vi "GatheringSerialPortNames.vi"() -> (1 "name":string)   [LabVIEW 2016]
panel:
  in  "done":bool
  in  "Name":string
  in  "Refresh":bool
  in  "Name It":bool
  in  "Ports":i32(listbox)
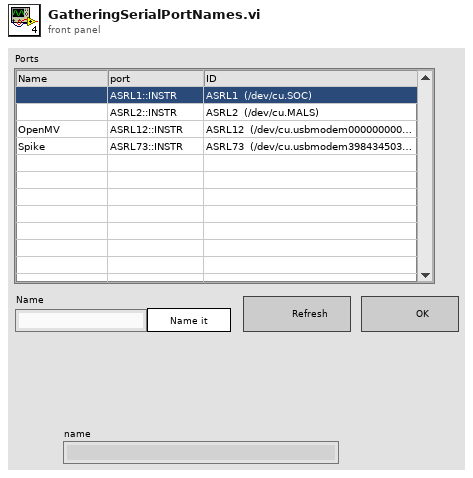
[diagram p1: front panel]
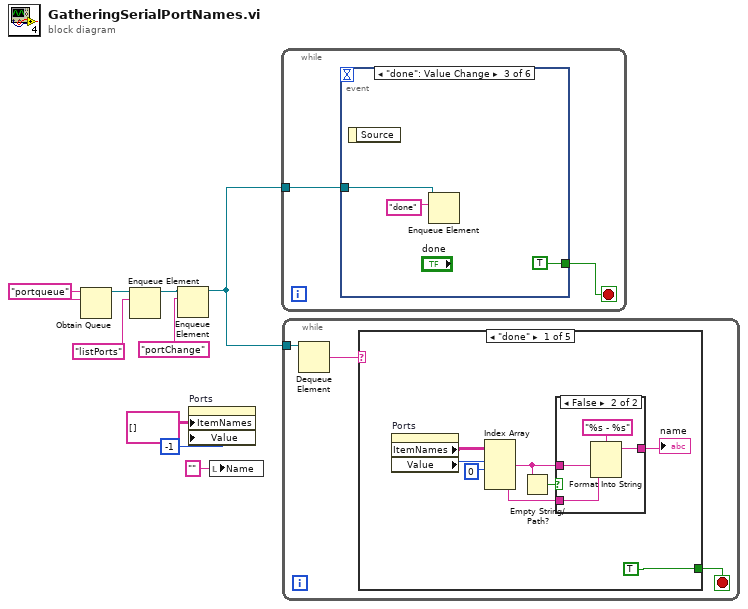
[diagram p0: block diagram]
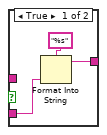
[diagram p2: hidden frame]
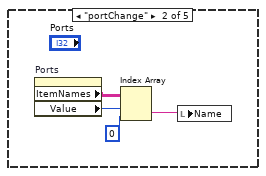
[diagram p3: hidden frame]
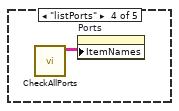
[diagram p5: hidden frame]
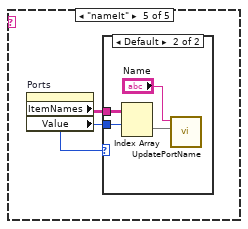
[diagram p6: hidden frame]
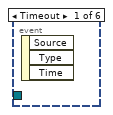
[diagram p8: hidden frame]
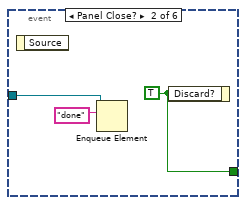
[diagram p9: hidden frame]
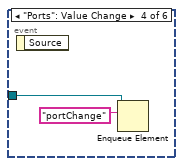
[diagram p10: hidden frame]
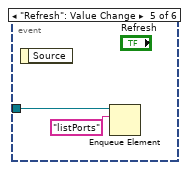
[diagram p11: hidden frame]
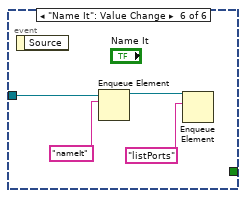
[diagram p12: hidden frame]
diagram:
  w7 = "portqueue" ("name (unnamed)")
  n1 = Obtain Queue(name (unnamed)=w7, element data type=w7) -> (queue out=w9:refnum<queue>)  [unwired: 3 in, 2 out]
  n2 = Enqueue Element(queue=w9, element="listPorts") -> (queue out=w5:refnum<queue>)  [unwired: 2 in, 2 out]
  n3 = Enqueue Element(queue=w5, element="portChange") -> (queue out=w4:refnum<queue>)  [unwired: 2 in, 2 out]
  n4 = property on="Ports" class="MCListbox (strict)"("ItemNames"=string[][] [] ("Item Names"), "Value"=-1 ("Ports")) -> ()  [unwired: 2 in, 2 out]
  n5 = local write "Name"("" ("Name")) -> ()
  n6 = while {
    tunnel: w4 -> [w10]
    stop <- w11 stop-if-true
    n7 = event shown="[2] \"done\": Value Change" {
      selector: _ -> [_ _ _ _ _ _]
      dyn-events: _ -> [_ _ _ _ _ _]
      timeout: _ -> [_ _ _ _ _ _]
      tunnel: [_ w14 TRUE ("Discard?") _ _ _] -> w11
      tunnel: w10 -> [_ w12 w16 w18 w20 w23]
      event Timeout {
        n8 = event-data() -> ()  [unwired: 1 in, 3 out]
      }
      event Panel Close? {
        w14 = TRUE ("Discard?")
        n9 = event-data() -> ()  [unwired: 1 in, 1 out]
        n10 = Enqueue Element(queue=w12, element="done") -> ()  [unwired: 2 in, 3 out]
        n11 = event-data("Discard?"=w14) -> ()  [unwired: 1 in, 1 out]
      }
      event "done": Value Change {
        n12 = event-data() -> ()  [unwired: 1 in, 1 out]
        n13 = Enqueue Element(queue=w16, element="done") -> ()  [unwired: 2 in, 3 out]
      }
      event "Ports": Value Change {
        n14 = event-data() -> ()  [unwired: 1 in, 1 out]
        n15 = Enqueue Element(queue=w18, element="portChange") -> ()  [unwired: 2 in, 3 out]
      }
      event "Refresh": Value Change {
        n16 = event-data() -> ()  [unwired: 1 in, 1 out]
        n17 = Enqueue Element(queue=w20, element="listPorts") -> ()  [unwired: 2 in, 3 out]
      }
      event "Name It": Value Change {
        n18 = event-data() -> ()  [unwired: 1 in, 1 out]
        n19 = Enqueue Element(queue=w23, element="nameIt") -> (queue out=w22:refnum<queue>)  [unwired: 2 in, 2 out]
        n20 = Enqueue Element(queue=w22, element="listPorts") -> ()  [unwired: 2 in, 3 out]
      }
    }
  }
  n21 = while {
    tunnel: w4 -> [w28]
    stop <- w26 stop-if-true
    n22 = Dequeue Element(queue=w28) -> (element=w27:string)  [unwired: 2 in, 3 out]
    n23 = case shown="\"done\"" w27 {
      tunnel: [TRUE _ _ _ _] -> w26
      frame "done" {
        n24 = property on="Ports" class="MCListbox (strict)"() -> ("ItemNames"=w35:string[][], "Value"=w34:i32)  [unwired: 2 in, 2 out]
        n25 = Index Array(array=w35, index (row) #1=w34, index (col) #1=0 ("disabled index (col)")) -> (element #1=w30:string, element #2=w29:string)  [unwired: 2 in]
        n26 = Empty String/Path?(string/path=w30) -> (empty?=w33:bool)
        n27 = case shown="False" w33 {
          tunnel: w29 -> [w37 w42]
          tunnel: [w38 w41] -> w32
          tunnel: w30 -> [_ w40]
          frame True {
            n28 = Format Into String(format string="%s", w37) -> (resulting string=w38:string)  [unwired: 2 in, 1 out]
          }
          frame False {
            n29 = Format Into String(format string="%s - %s", w40, w42) -> (resulting string=w41:string)  [unwired: 2 in, 1 out]
          }
        }
        "name" <- w32
      }
      frame "portChange" {
        n30 = property on="Ports" class="MCListbox (strict)"() -> ("ItemNames"=w47:string[][], "Value"=w45:i32)  [unwired: 2 in, 2 out]
        n31 = Index Array(array=w47, index (row)=w45, index (col)=0 ("disabled index (col)")) -> (element=w44:string)
        n32 = local write "Name"(w44) -> ()
      }
      frame Default {
      }
      frame "listPorts" {
        n33 = call "CheckAllPorts.vi"() -> ("Ports"=w48:string[][])  [unwired: 11 in]
        n34 = property on="Ports" class="MCListbox (strict)"("ItemNames"=w48) -> ()  [unwired: 2 in, 2 out]
      }
      frame "nameIt" {
        n35 = property on="Ports" class="MCListbox (strict)"() -> ("ItemNames"=w50:string[][], "Value"=w49:i32)  [unwired: 2 in, 2 out]
        n36 = case shown="Default" w49 {
          tunnel: w50 -> [_ w54]
          tunnel: w49 -> [_ w53]
          frame -1 {
          }
          frame Default {
            n37 = Index Array(array=w54, index (row)=w53) -> (element=w52:string[])  [unwired: 1 in]
            n38 = call "UpdatePortName.vi"("ItemNames"=w52, "Name"="Name") -> ()  [unwired: 10 in]
          }
        }
      }
    }
  }
